vi "Load Vorbis.vi"(8 "error in (no error)":errorcluster, 11 "Path":path) -> (0 "error out":errorcluster, 1 "data":waveform(i16)[](array[waveform]), 2 "Sample Rate (Hz)":i32, 3 "Channels":i32, 5 "Length (Samples)":i32)   [LabVIEW 2019, in "Audio File Input.lvlib"]
doc: "Loads an Ogg Vorbis file from disk.\n\n<b>Priority:</b> Background priority (lowest)"
uses:
  Audio File Input.lvlib
  external/audio_decoder_library_wrapper/lib/audio_decoder_library_wrapper.dll
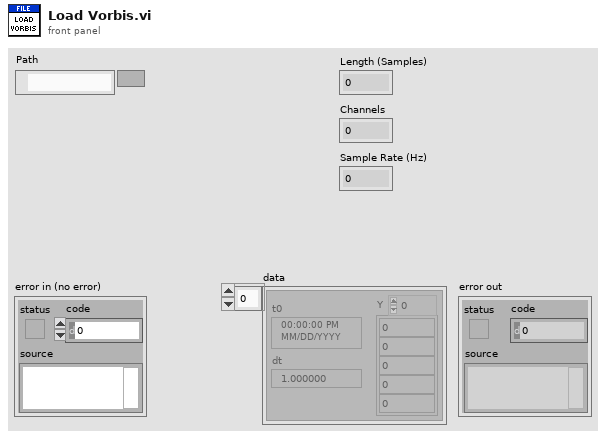
[diagram p1: front panel]
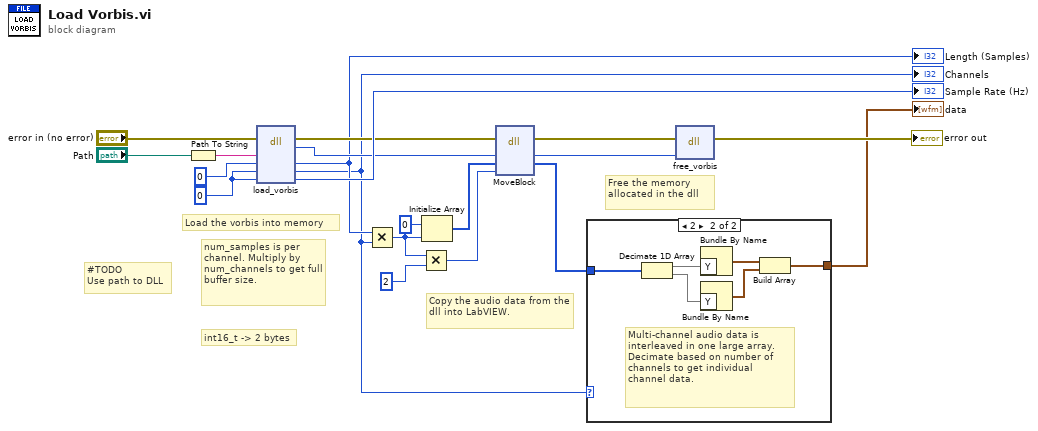
[diagram p0: block diagram]
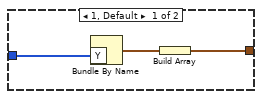
[diagram p2: hidden frame]
diagram:
  w15 = u32 0 ("num_samples")
  # "num_samples is per channel. Multiply by num_channels to get full buffer size."
  # "#TODO\nUse path to DLL"
  # "Free the memory allocated in the dll"
  # "Copy the audio data from the dll into LabVIEW."
  # "Load the vorbis into memory"
  # "int16_t -> 2 bytes"
  n1 = Path To String(path="Path") -> (string=w16:string)
  n2 = dll-call lib="C:/github/dataflowg/dataflow-dj/external/audio_decoder_library_wrapper/lib/audio_decoder_library_wrapper.dll" fn="load_vorbis"(error in="error in (no error)", "file_name"=w16, "num_samples"=u64 0, "channels"=w15, "sample_rate"=w15) -> (error out=w11:errorcluster, "return type"=w13:i64, "num_samples"=w3:i32, "channels"=w2:i32, "sample_rate"=→"Sample Rate (Hz)":i32)  [unwired: 3 in, 1 out]
  "Length (Samples)" <- w3
  "Channels" <- w2
  n3 = Multiply(x=w3, y=w2) -> (x*y=w1:i32)
  n4 = Multiply(x=w1, y=2) -> (x*y=w9:i32)
  n5 = Initialize Array(i16 0 ("num_samples"), w1) -> (w12:i16[])
  n6 = dll-call lib="LabVIEW" fn="MoveBlock"(error in=w11, "Address (Pointer)"=w13, "Destination"=w12, "Size"=w9) -> (error out=w7:errorcluster, "Address (Pointer)"=w8:i64, "Destination"=w6:i16[])  [unwired: 4 in, 1 out]
  n7 = case shown="2" w2 {
    tunnel: w6 -> [w23 w29]
    tunnel: [w22 w24] -> w4
    frame 1, Default {
      n8 = Bundle By Name("Y"=w23) -> (w21:waveform(i16))  [unwired: 1 in]
      n9 = Build Array(w21) -> (w22:waveform(i16)[])
    }
    frame 2 {
      # "Multi-channel audio data is interleaved in one large array. Decimate based on number of channels to get individual channel data."
      n10 = Decimate 1D Array(w29) -> (w28:i16[], w27:i16[])
      n11 = Bundle By Name("Y"=w28) -> (w26:waveform(i16))  [unwired: 1 in]
      n12 = Bundle By Name("Y"=w27) -> (w25:waveform(i16))  [unwired: 1 in]
      n13 = Build Array(w26, w25) -> (w24:waveform(i16)[])
    }
  }
  "data" <- w4
  n14 = dll-call lib="C:/github/dataflowg/dataflow-dj/external/audio_decoder_library_wrapper/lib/audio_decoder_library_wrapper.dll" fn="free_vorbis"(error in=w7, "Address (Pointer)"=w8) -> (error out=→"error out":errorcluster)  [unwired: 4 in, 1 out]
